vi "Find Devices.vi"(0 "DeviceCount":i32, 1 "error in (no error)":errorcluster) -> (2 "DeviceCount out":i32, 3 "function return":i32, 4 "error out":errorcluster)   [LabVIEW 2017, in "MCM3000.lvlib"]
doc: "long FindDevices(long &DeviceCount);"
uses:
  MCM3000.lvlib
  ThorMCM3000.dll
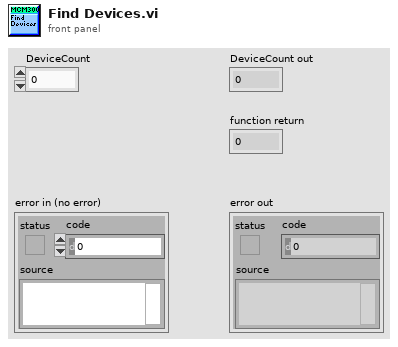
[diagram p1: front panel]
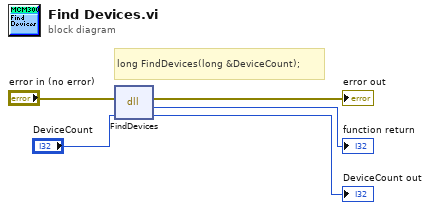
[diagram p0: block diagram]
diagram:
  # "long FindDevices(long &DeviceCount);"
  n1 = dll-call lib="D:/ChipScope Control/LabVIEW-control/Stage subVIs/MCM3000/LabVIEW/inc/ThorMCM3000.*" fn="FindDevices"(error in="error in (no error)", "DeviceCount"="DeviceCount") -> (error out=→"error out":errorcluster, →"function return":i32, "DeviceCount"=→"DeviceCount out":i32)  [unwired: 2 in, 1 out]
